vi "Bar Graph Test Program.vi"() -> ()   [LabVIEW 2014]
uses:
  <vilib>/Utility/miscctls.llb/LVPoint32TypeDef.ctl
panel:
  in  "Ring":u16(ring)
  in  "Multicolumn Listbox":i32(listbox)
  in  "stop":bool
  out "Y":dbl
  out "Coords":T1
  out "Stacked Bar Plots":dbl[][](graph)
  out "XY Graph":cluster{dbl[], dbl[]}[](graph)
  out "Annual Report 2":cluster{dbl[], dbl[]}[](graph)
  in  "Table":string[][](table)=[["34", "74", "23", "35", "23", "26", "74", "74", "21", "39", "61", "83"], ["73", "24", "75", "87", "42", "34", "35", "76", "52", "43", "43", "3"], ["36", "25", "12", "34", "24", "74", "73", "54", "88", "64", "90", "62"]]
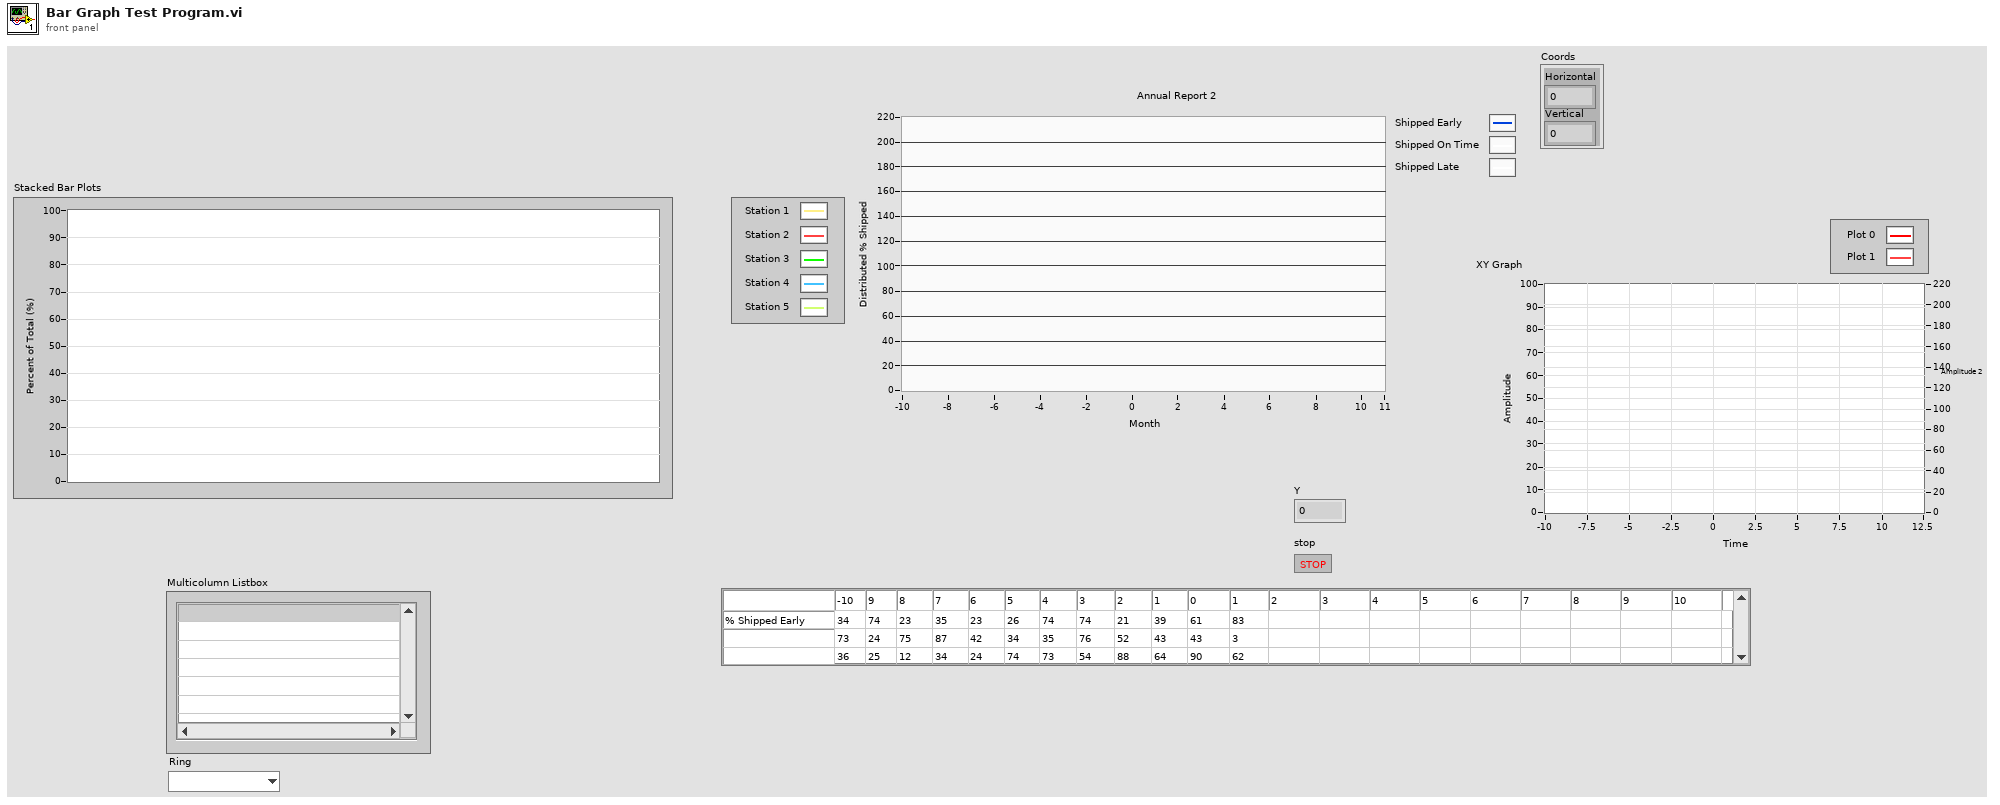
[diagram p1: front panel]
types:
  T1 = typedef "LVPoint32TypeDef.ctl" = cluster{"Horizontal":i32, "Vertical":i32}
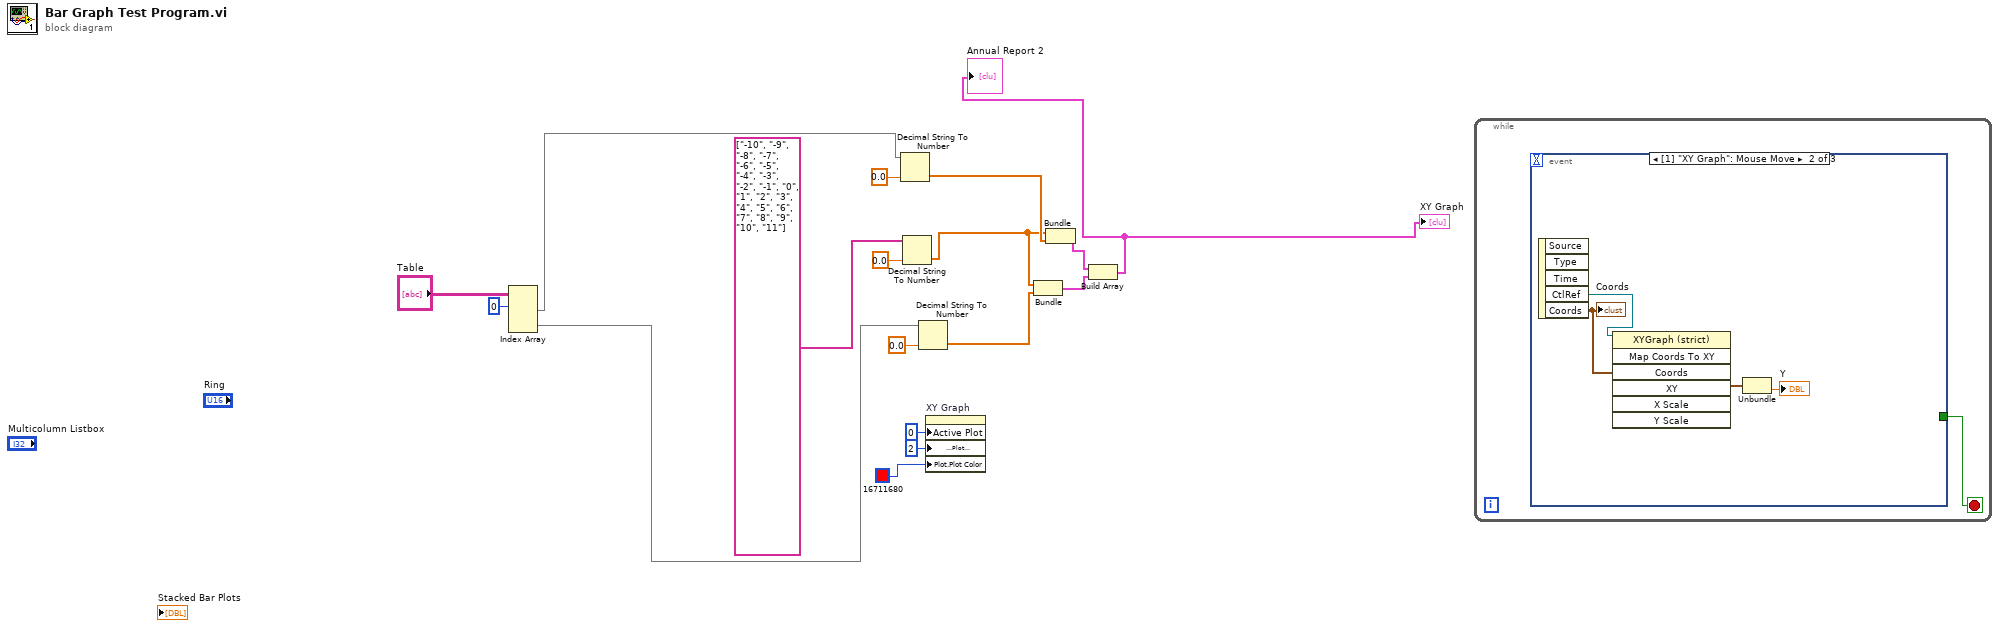
[diagram p0: block diagram]
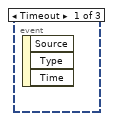
[diagram p2: hidden frame]
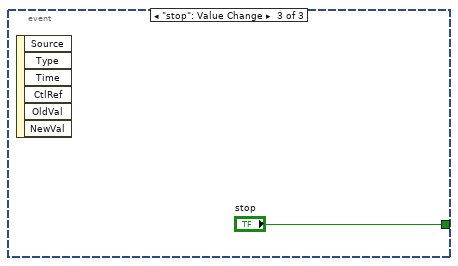
[diagram p3: hidden frame]
diagram:
  n1 = Index Array(array="Table", index (row) #1=0 ("index (row)")) -> (element #1=w14:string[], element #2=w5:string[])  [unwired: 3 in]
  n2 = Decimal String To Number(string=w14, default (0L)=0.0) -> (number=w11:dbl[])  [unwired: 1 in, 1 out]
  n3 = Decimal String To Number(string=string[] ["-10", "-9", "-8", "-7", "-6", "-5", "-4", "-3", "-2", "-1", "0", "1", "2", "3", "4", "5", "6", "7", "8", "9", "10", "11"], default (0L)=0.0) -> (number=w4:dbl[])  [unwired: 1 in, 1 out]
  n4 = Decimal String To Number(string=w5, default (0L)=0.0) -> (number=w3:dbl[])  [unwired: 1 in, 1 out]
  n5 = property on="XY Graph" class="XYGraph (strict)"("Active Plot"=u32 0, "Plot.Plot Interpolation"=u8 2, "Plot.Plot Color"=u32 16711680) -> ()  [unwired: 2 in, 2 out]
  n6 = Bundle(w4, w3) -> (w2:cluster{dbl[], dbl[]})  [unwired: 1 in]
  n7 = Bundle(w4, w11) -> (w7:cluster{dbl[], dbl[]})  [unwired: 1 in]
  n8 = Build Array(w7, w2) -> (→"Annual Report 2" →"XY Graph":cluster{dbl[], dbl[]}[])
  n9 = while {
    stop <- w18 stop-if-true
    n10 = event shown="[1] \"XY Graph\": Mouse Move" {
      selector: _ -> [_ _ _]
      dyn-events: _ -> [_ _ _]
      timeout: _ -> [_ _ _]
      tunnel: [_ _ "stop"] -> w18
      event Timeout {
        n11 = event-data() -> ()  [unwired: 1 in, 3 out]
      }
      event "XY Graph": Mouse Move {
        n12 = event-data() -> ("CtlRef"=w19:refnum<vi>, "Coords"=w22:T1)  [unwired: 1 in, 3 out]
        "Coords" <- w22
        n13 = invoke class="XYGraph (strict)" method="Map Coords To XY"(reference=w19, "Coords"=w22) -> ("XY"=w21:cluster{"X":dbl, "Y":dbl})  [unwired: 5 in, 6 out]
        n14 = Unbundle(w21) -> ("Y"=→"Y":dbl)  [unwired: 1 out]
      }
      event "stop": Value Change {
        n15 = event-data() -> ()  [unwired: 1 in, 6 out]
      }
    }
  }
